vi "Recalculation_Monitor.vi"(0 "Alpha":dbl(slide)=0.17500000000000002 step=0.005 scale=0.0..1.0, 1 "Message 1":string="Lorem ipsum dolor sit amet, consetetur sadipscing elitr, sed diam nonumy eirmod tempor invidunt ut labore et dolore magna aliquyam erat, sed diam volu", 2 "Message 2":string="ptua. At vero eos et accusam et justo duo dolores et ea rebum. Stet clita kasd gubergren, no sea takimata sanctus est Lorem ipsum dolor sit amet. Lore", 3 "Alpha old":dbl(slide)=0.17500000000000002 step=0.005 scale=0.0..1.0, 4 "Message 1 old":string="Lorem ipsum dolor sit amet, consetetur sadipscing elitr, sed diam nonumy eirmod tempor invidunt ut labore et dolore magna aliquyam erat, sed diam volu", 5 "Message 2 old":string="ptua. At vero eos et accusam et justo duo dolores et ea rebum. Stet clita kasd gubergren, no sea takimata sanctus est Lorem ipsum dolor sit amet. Lore") -> (14 "Recalculate?":bool, 15 "Recalculate SIG":bool, 16 "Recalculate OFDM":bool)   [LabVIEW 2022 SP3]
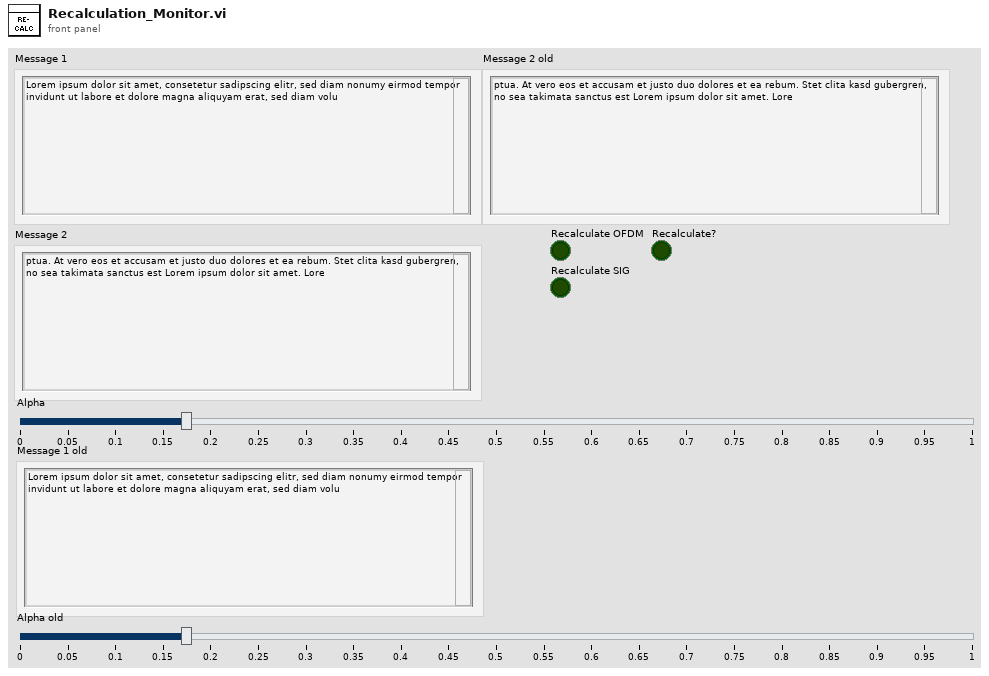
[diagram p1: front panel]
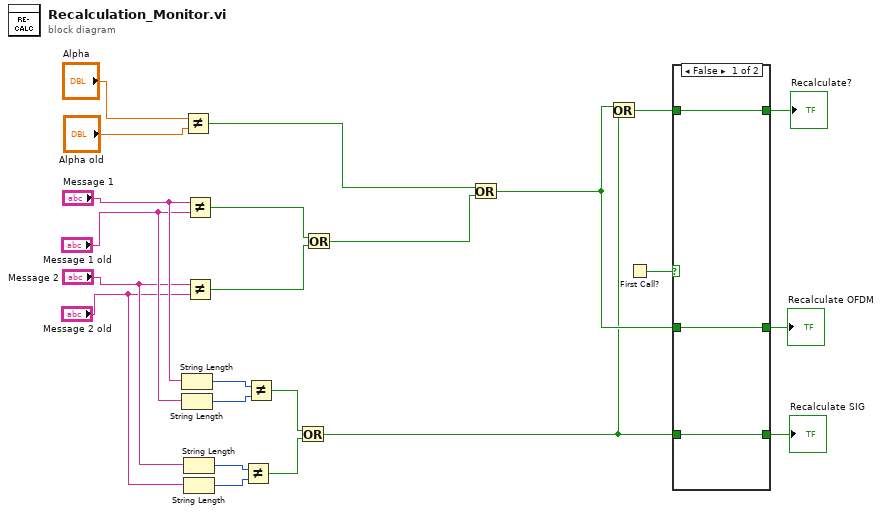
[diagram p0: block diagram]
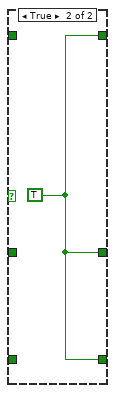
[diagram p2: hidden frame]
diagram:
  n1 = String Length(string="Message 1") -> (length=w15:i32)
  n2 = String Length(string="Message 1 old") -> (length=w14:i32)
  n3 = Not Equal?(x="Alpha", y="Alpha old") -> (x != y?=w9:bool)
  n4 = String Length(string="Message 2") -> (length=w13:i32)
  n5 = String Length(string="Message 2 old") -> (length=w12:i32)
  n6 = Not Equal?(x="Message 1", y="Message 1 old") -> (x != y?=w21:bool)
  n7 = Not Equal?(x="Message 2", y="Message 2 old") -> (x != y?=w20:bool)
  n8 = Not Equal?(x=w13, y=w12) -> (x != y?=w10:bool)
  n9 = Not Equal?(x=w15, y=w14) -> (x != y?=w11:bool)
  n10 = Or(x=w11, y=w10) -> (x .or. y?=w1:bool)
  n11 = Or(x=w21, y=w20) -> (x .or. y?=w8:bool)
  n12 = Or(x=w9, y=w8) -> (x .or. y?=w2:bool)
  n13 = Or(x=w2, y=w1) -> (x .or. y?=w3:bool)
  n14 = First Call?() -> (First Call?: T/F=w7:bool)
  n15 = case shown="False" w7 {
    tunnel: [w24 w27] -> w6
    tunnel: [w25 w27] -> w5
    tunnel: [w26 w27] -> w4
    tunnel: w3 -> [w26 _]
    tunnel: w2 -> [w25 _]
    tunnel: w1 -> [w24 _]
    frame False {
    }
    frame True {
      w27 = TRUE
    }
  }
  "Recalculate OFDM" <- w5
  "Recalculate SIG" <- w6
  "Recalculate?" <- w4
